vi "myRIO_BRig_Host_stateIdxList_wrong.vi"() -> (1 "output_min_wrong":u16=32, 3 "output_max_wrong":u16=35)   [LabVIEW 2014]
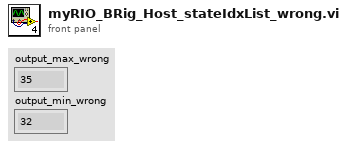
[diagram p1: front panel]
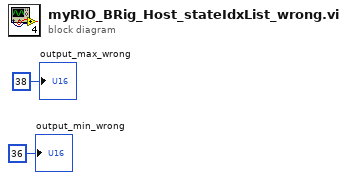
[diagram p0: block diagram]
diagram:
  "output_max_wrong" <- u16 38
  "output_min_wrong" <- u16 36
